vi "updateDataOut.vi"(8 "error in (no error)":errorcluster) -> (0 "error out":errorcluster)   [LabVIEW 2017]
uses:
  TypeDefs/UDPListenFGVCtrl.ctl
  TypeDefs/dataOut.ctl
  TypeDefs/dataFGVState.ctl
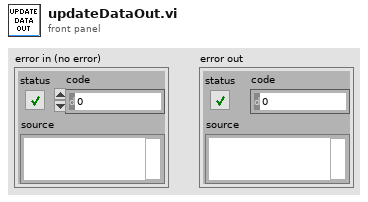
[diagram p1: front panel]
types:
  T1 = typedef "dataFGVState.ctl" = enum16{"init", "write data out", "read data out", "write data in", "read data in"}
  T2 = typedef "UDPListenFGVCtrl.ctl" = enum16{"Read", "Write"}
  T3 = typedef "dataOut.ctl" = cluster{"X0pos":dbl, "Y0pos":dbl, "Z0pos":dbl, "Fx":dbl, "Fy":dbl, "Fz":dbl, "Encoder1":i32, "Encoder2":i32, "Pot1":dbl, "Pot2":dbl, "Theta0":dbl, "Theta1":dbl, "X1pos":dbl, "Y1pos":dbl, "Z1pos":dbl, "X2pos":dbl, "Y2pos":dbl, "Z2pos":dbl, "ErrorOccurred":bool}
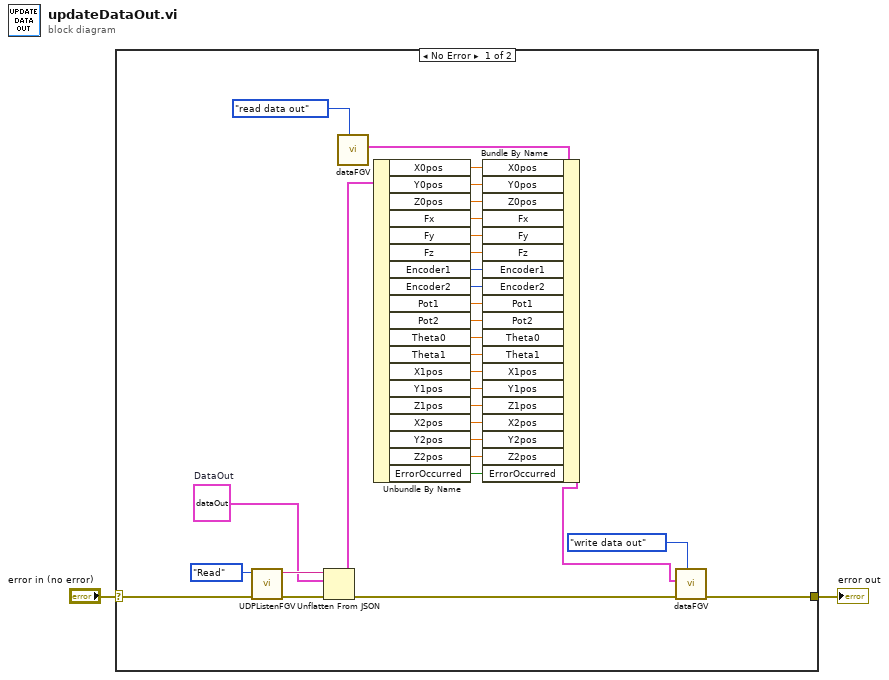
[diagram p0: block diagram]
diagram:
  n1 = case shown="No Error" "error in (no error)" {
    selector: "error in (no error)" -> [w27 w34]
    tunnel: [w26 w34] -> w1
    frame No Error {
      w31 = T3 {"X0pos"=0.0, "Y0pos"=0.0, "Z0pos"=0.0, "Fx"=0.0, "Fy"=0.0, "Fz"=0.0, "Encoder1"=0, "Encoder2"=0, "Pot1"=0.0, "Pot2"=0.0, "Theta0"=0.0, "Theta1"=0.0, "X1pos"=0.0, "Y1pos"=0.0, "Z1pos"=0.0, "X2pos"=0.0, "Y2pos"=0.0, "Z2pos"=0.0, "ErrorOccurred"=FALSE}  # DataOut
      n2 = call "UDPListenFGV.vi"("error in (no error)"=w27, "Enum"=UDPListenFGVCtrl."Read") -> ("error out"=w30:errorcluster, "Read Data"=w32:string)  [unwired: 8 in]
      n3 = Unflatten From JSON(JSON string=w32, type and defaults=w31, error in (no error)=w30) -> (value=w23:T3, error out=w28:errorcluster)  [unwired: 4 in]
      n4 = call "dataFGV.vi"("Enum"=dataFGVState."read data out") -> ("DataOut"=w24:T3)  [unwired: 8 in, 2 out]
      n5 = Unbundle By Name(w23) -> ("X0pos"=w4:dbl, "Y0pos"=w5:dbl, "Z0pos"=w6:dbl, "Fx"=w7:dbl, "Fy"=w8:dbl, "Fz"=w9:dbl, "Encoder1"=w10:i32, "Encoder2"=w11:i32, "Pot1"=w12:dbl, "Pot2"=w13:dbl, "Theta0"=w14:dbl, "Theta1"=w15:dbl, "X1pos"=w16:dbl, "Y1pos"=w17:dbl, "Z1pos"=w18:dbl, "X2pos"=w19:dbl, "Y2pos"=w20:dbl, "Z2pos"=w21:dbl, "ErrorOccurred"=w22:bool)
      n6 = Bundle By Name(cluster=w24, "X0pos"=w4, "Y0pos"=w5, "Z0pos"=w6, "Fx"=w7, "Fy"=w8, "Fz"=w9, "Encoder1"=w10, "Encoder2"=w11, "Pot1"=w12, "Pot2"=w13, "Theta0"=w14, "Theta1"=w15, "X1pos"=w16, "Y1pos"=w17, "Z1pos"=w18, "X2pos"=w19, "Y2pos"=w20, "Z2pos"=w21, "ErrorOccurred"=w22) -> (w3:T3)
      n7 = call "dataFGV.vi"("Enum"=dataFGVState."write data out", "error in (no error)"=w28, "DataOut"=w3) -> ("error out"=w26:errorcluster)  [unwired: 6 in, 2 out]
    }
    frame Error {
    }
  }
  "error out" <- w1
